vi "產生圓.vi"() -> ()   [LabVIEW 2015]
panel:
  out "now":cluster{dbl[], dbl[]}(graph)
  out "XY Graph":cluster{dbl[], dbl[]}(graph)
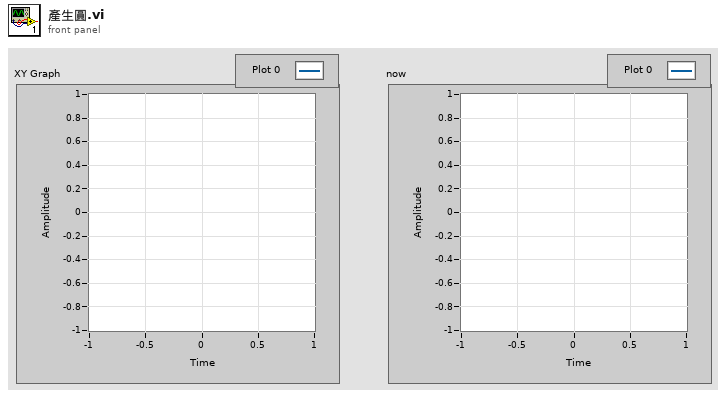
[diagram p1: front panel]
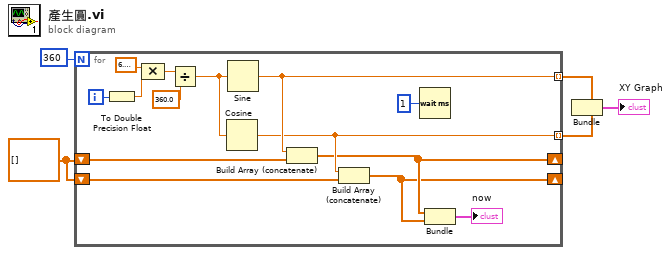
[diagram p0: block diagram]
diagram:
  w1 = dbl[] []
  n1 = for {
    N: 360 ("Numeric") -> [_]
    tunnel: [w11] -> w4 mode=indexing
    tunnel: [w10] -> w3 mode=indexing
    shift-right: [w6] -> _
    shift-left: w1 -> [w9]
    shift-right: [w7] -> _
    shift-left: w1 -> [w12]
    i -> [w18]
    n2 = To Double Precision Float(number=w18) -> (double precision float=w17:dbl)
    n3 = Compound Arithmetic op=MULTIPLY(6.283185307179586, w17) -> (w16:dbl)
    n4 = Divide(x=w16, y=360.0) -> (x/y=w14:dbl)
    n5 = Cosine(x=w14) -> (cos(x)=w10:dbl)
    n6 = Sine(x=w14) -> (sin(x)=w11:dbl)
    n7 = Build Array (concatenate)(w11, w12) -> (w7:dbl[])
    n8 = Build Array (concatenate)(w10, w9) -> (w6:dbl[])
    n9 = Wait (ms)(milliseconds to wait=u32 1) -> ()  [unwired: 1 out]
    n10 = Bundle(w7, w6) -> (→"now":cluster{dbl[], dbl[]})  [unwired: 1 in]
  }
  n11 = Bundle(w4, w3) -> (→"XY Graph":cluster{dbl[], dbl[]})  [unwired: 1 in]
